vi "Task 4 revisited.vi"() -> ()   [LabVIEW 2024]
panel:
  in  "V":dbl[](array[numeric])
  out "Array":dbl[][](array[numeric])
  in  "G":dbl[](array[numeric])
  in  "T":dbl[](array[numeric])
  in  "T":dbl
  in  "G":dbl
  out "I_ph":dbl
  out "I_sh":dbl
  out "I_0":dbl
  out "I_rs":dbl
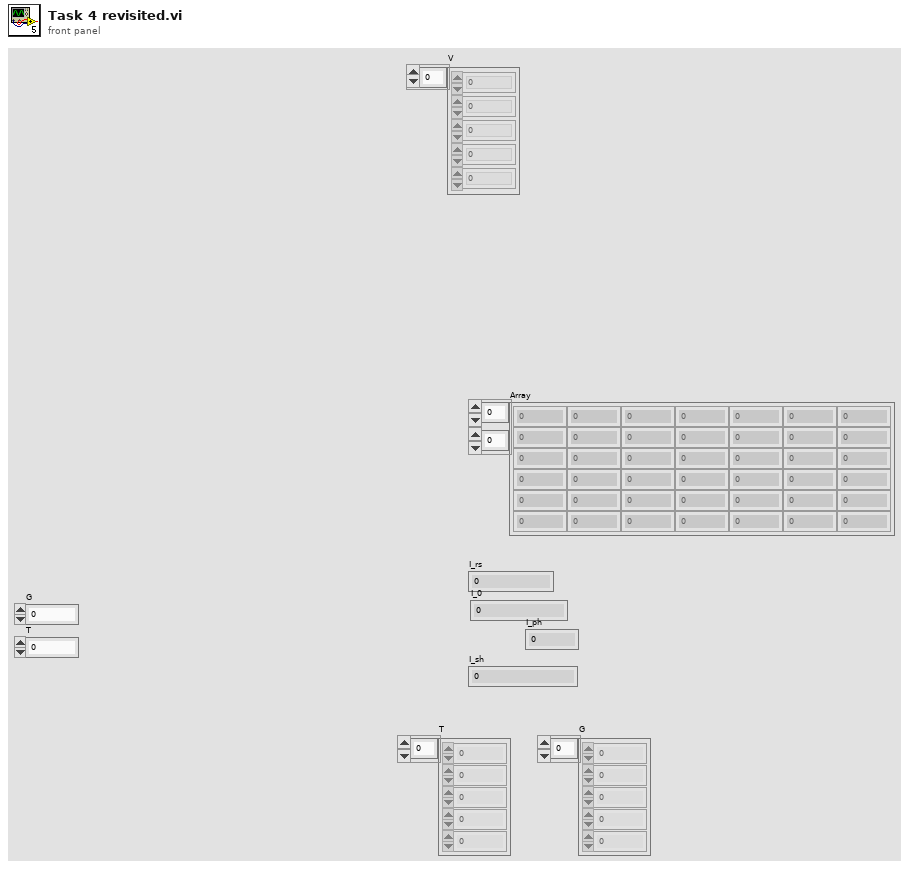
[diagram p1: front panel]
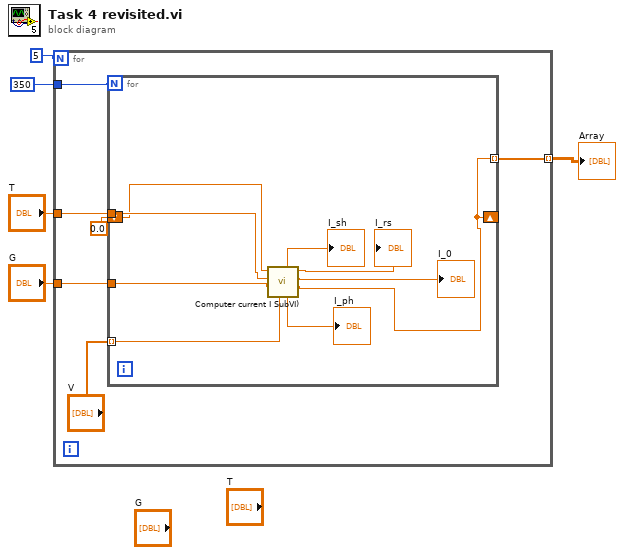
[diagram p0: block diagram]
diagram:
  n1 = for {
    N: 5 -> [_]
    tunnel: "G" -> [w11]
    tunnel: "T" -> [w10]
    tunnel: 350 -> [w9]
    tunnel: [w7] -> w1 mode=indexing
    n2 = for {
      N: w9 -> [_]
      tunnel: "V" -> [w12] mode=indexing
      tunnel: w11 -> [w15]
      tunnel: w10 -> [w16]
      shift-right: [w17] -> _
      shift-left: 0.0 ("I") -> [w14]
      tunnel: [w17] -> w7 mode=indexing
      n3 = call "Computer current I SubVI).vi"("V"=w12, "G"=w15, "T"=w16, "I_1"=w14) -> ("I"=w17:dbl, "I_0"=→"I_0":dbl, "I_rs"=→"I_rs":dbl, "I_ph"=→"I_ph":dbl, "I_sh"=→"I_sh":dbl)  [unwired: 3 in]
    }
  }
  "Array" <- w1
